vi "validate_and_push.vi"(8 "error in (no error)":errorcluster, 9 "values":dbl[](array[numeric]), 10 "timestamps_ns":u64[](array[numeric]), 11 "writer_handle":u64) -> (0 "error out":errorcluster)   [LabVIEW 2020, in "Nominal Streaming.lvlib" / "Channel.lvclass"]
uses:
  Channel.lvclass
  Channel.lvclass/Channel.ctl
  bin/lib_nominal-streaming-lv_64.dll
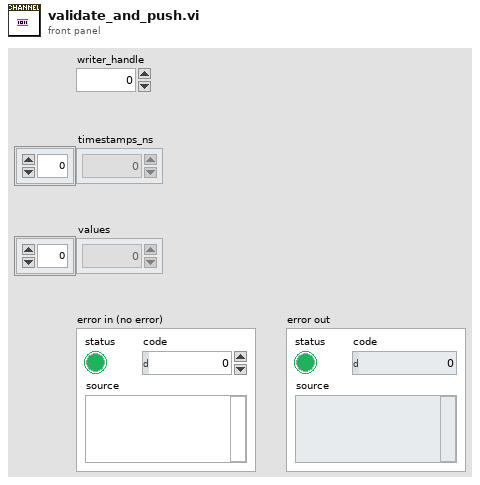
[diagram p1: front panel]
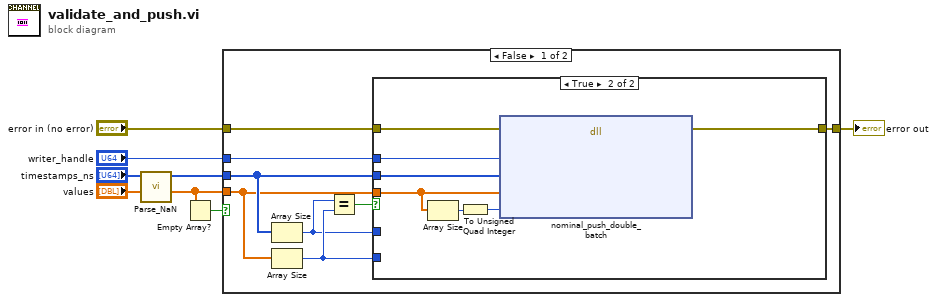
[diagram p0: block diagram]
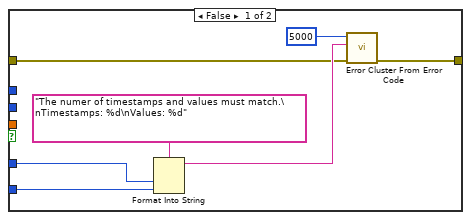
[diagram p2: hidden frame]
diagram:
  n1 = call "Parse_NaN.vi"("values"="values", "timestamps_ns"="timestamps_ns") -> ("Filtered Values"=w2:dbl[], "Filtered Timestamps"=w3:u64[])  [unwired: 8 in]
  n2 = Empty Array?(array=w2) -> (empty?=w1:bool)
  n3 = case shown="False" w1 {
    tunnel: "error in (no error)" -> [w16 w31]
    tunnel: "writer_handle" -> [w15 _]
    tunnel: [w14 w31] -> w6
    tunnel: w3 -> [w13 _]
    tunnel: w2 -> [w12 _]
    frame False {
      n4 = Array Size(array=w13) -> (size(s)=w9:i32)
      n5 = Array Size(array=w12) -> (size(s)=w10:i32)
      n6 = Equal?(x=w9, y=w10) -> (x = y?=w11:bool)
      n7 = case shown="True" w11 {
        tunnel: w16 -> [w18 w29]
        tunnel: w15 -> [_ w28]
        tunnel: [w17 w27] -> w14
        tunnel: w13 -> [_ w25]
        tunnel: w12 -> [_ w24]
        tunnel: w10 -> [w21 _]
        tunnel: w9 -> [w20 _]
        frame False {
          n8 = Format Into String(format string="The numer of timestamps and values must match.\nTimestamps: %d\nValues: %d" ("error message (\"\")"), w20, w21) -> (resulting string=w19:string)  [unwired: 2 in, 1 out]
          n9 = call <vilib>:"Error Cluster From Error Code.vi"("error in (no error)"=w18, "error message (\"\")"=w19, "error code (0)"=5000) -> ("error out"=w17:errorcluster)  [unwired: 6 in]
        }
        frame True {
          n10 = Array Size(array=w24) -> (size(s)=w30:i32)
          n11 = To Unsigned Quad Integer(1:w30) -> (0:w26:u64)
          n12 = dll-call lib="C:/code/nominal-streaming-labview-ffi/lv_src/bin/lib_nominal-streaming-lv_*.*" fn="nominal_push_double_batch"(error in=w29, "writer_handle"=w28, "timestamps_ns"=w25, "values"=w24, "count"=w26) -> (error out=w27:errorcluster)  [unwired: 7 in, 1 out]
        }
      }
    }
    frame True {
    }
  }
  "error out" <- w6
